vi "4_1.vi"() -> ()   [LabVIEW 2012]
panel:
  in  "Boolean":bool
  out "Array":dbl[](array[numeric])
  in  "x":i32
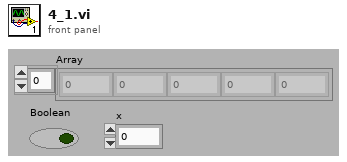
[diagram p1: front panel]
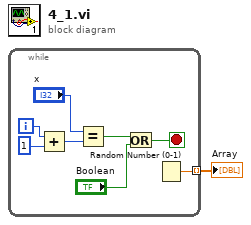
[diagram p0: block diagram]
diagram:
  n1 = while {
    tunnel: [w9] -> w1 mode=indexing
    i -> [w6]
    stop <- w2 stop-if-true
    n2 = Add(x=w6, y=1) -> (x+y=w7:i32)
    n3 = Equal?(x="x", y=w7) -> (x = y?=w4:bool)
    n4 = Or(x=w4, y="Boolean") -> (x .or. y?=w2:bool)
    n5 = Random Number (0-1)() -> (number: 0 to 1=w9:dbl)
  }
  "Array" <- w1
